vi "ZUP Write Voltage Level.vi"(8 "error in (no error)":errorcluster, 10 "Voltage":dbl, 11 "VISA resource name":refnum<visa-resource-name>) -> (0 "error out":errorcluster, 2 "Received Message":string, 3 "VISA OUT":refnum<visa-resource-name>)   [LabVIEW 2018]
doc: "Requests the ZUP power supply to set the output voltage to a value specified by the user"
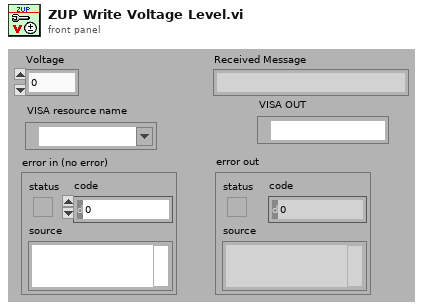
[diagram p1: front panel]
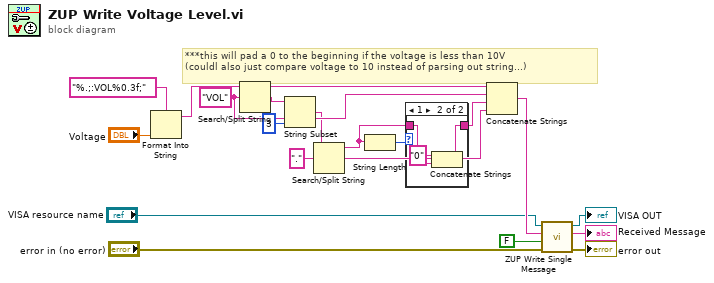
[diagram p0: block diagram]
diagram:
  w13 = "VOL" ("search string/char (-)")
  # "***this will pad a 0 to the beginning if the voltage is less than 10V\n(couldl also just compare voltage to 10 instead of parsing out string...)"
  n1 = Format Into String(format string="%.;:VOL%0.3f;" ("Command Out"), "Voltage") -> (resulting string=w5:string)  [unwired: 2 in, 1 out]
  n2 = Search/Split String(string=w5, search string/char (-)=w13) -> (substring before match=w14:string, match + rest of string=w12:string)  [unwired: 1 in, 1 out]
  n3 = String Subset(string=w12, offset (0)=3) -> (substring=w10:string)  [unwired: 1 in]
  n4 = Search/Split String(string=w10, search string/char (-)=".") -> (substring before match=w6:string, match + rest of string=w9:string)  [unwired: 1 in, 1 out]
  n5 = String Length(string=w6) -> (length=w8:i32)
  n6 = case shown="1" w8 {
    tunnel: [w21 w22] -> w7
    tunnel: w6 -> [w21 w24]
    frame 2, Default {
    }
    frame 1 {
      n7 = Concatenate Strings("0" ("string"), w24) -> (w22:string)
    }
  }
  n8 = Concatenate Strings(w14, w13, w7, w9) -> (w4:string)
  n9 = call "ZUP Write Single Message.vi"("error in (no error)"="error in (no error)", "Read Response"=FALSE, "Command Out"=w4, "VISA resource name"="VISA resource name") -> ("error out"=→"error out":errorcluster, "Received Message"=→"Received Message":string, "VISA OUT"=→"VISA OUT":refnum<visa-resource-name>)  [unwired: 4 in, 1 out]
